vi "buffer_get.vi"(0 "reference in":refnum<class "OSA.lvclass">, 5 "error in (no error)":errorcluster) -> (13 "spectrum X, (wavenr/cm)":sgl[](array[numeric]), 14 "reference out":refnum<class "OSA.lvclass">, 15 "interferogram (16bit)":sgl[](array[numeric]), 16 "interferogram prop":T3 {"contrast" format="%.2f"; "OPDmax (cm)" format="%.2f"; "OPDmin (cm)" format="%.2f"; "peakToPeak position (cm)" format="%.2f"; "peakToPeak, (counts)" format="%.2f"; "X max (cm)" format="%.2f"; "X min (cm)" format="%.2f"}, 17 "spectrum Y (mW)":sgl[](array[numeric]), 18 "spectrum properties":T2, 19 "error out":errorcluster)   [LabVIEW 2010, in "OSA.lvclass"]
doc: "This vi will read data from a labview interferogram and spectrum buffer. The buffer contains only the latest acquired interferogram and spectrum. Use the trace vis to simultaneously handle several data sets.\n\nInterferogram X data unit: cm\nInterferogram Y data unit: ADC counts, (see specs for nr of bits).\nSpectrum X data unit: /cm\nSpectrum Y data unit: mW\n\nFor some OSA, the Spectrum X array will only contain two values; x-min and max. This is indicated by the X VAL OPTION spectrum property (cluster).\n\nSee converter vis to obtain other units, (Modules Unit Conversion in FTSLib help).\n\nTransfer trace data to labview buffer with trace_toLVBuffer.vi."
uses:
  OSA.lvclass
  typeDef/interferogram_properties.ctl
  typeDef/xVal_option.ctl
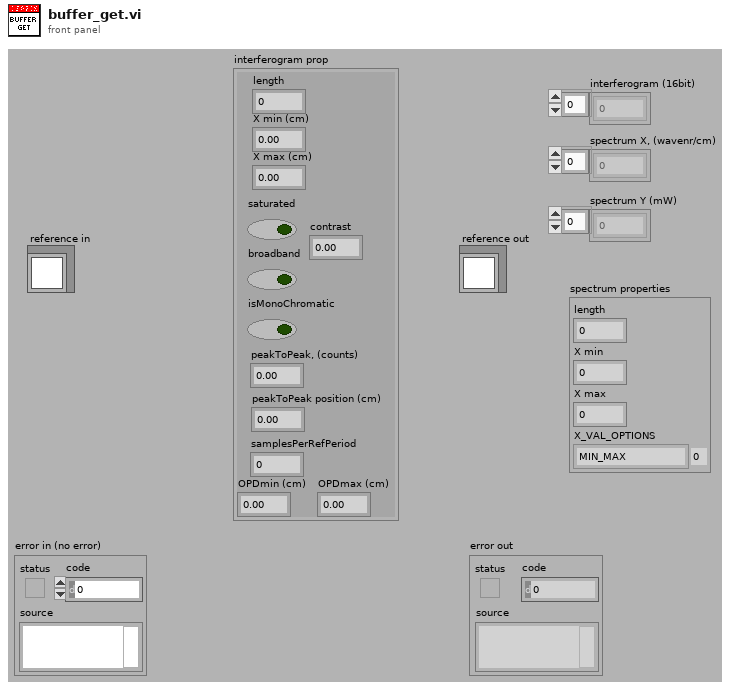
[diagram p1: front panel]
types:
  T1 = typedef "OSA.lvclass/xVal_option.ctl" = enum16{"MIN_MAX", "ARRAY"}
  T2 = cluster{"length":u32, "X min":sgl, "X max":sgl, "X_VAL_OPTIONS":T1}
  T3 = typedef "OSA.lvclass/interferogram_properties.ctl" = cluster{"length":u32, "X min (cm)":sgl, "X max (cm)":sgl, "saturated":bool, "broadband":bool, "isMonoChromatic":bool, "peakToPeak, (counts)":dbl, "peakToPeak position (cm)":dbl, "samplesPerRefPeriod":i32, "OPDmin (cm)":sgl, "OPDmax (cm)":sgl, "contrast":dbl}
  T4 = enum16{"get", "init", "set interferogram", "set spectrum", "cleanUp"}
  T5 = typedef "OSA.lvclass/spectrum_properties.ctl" = cluster{"length":u32, "X min":sgl, "X max":sgl, "X_VAL_OPTIONS":T1}
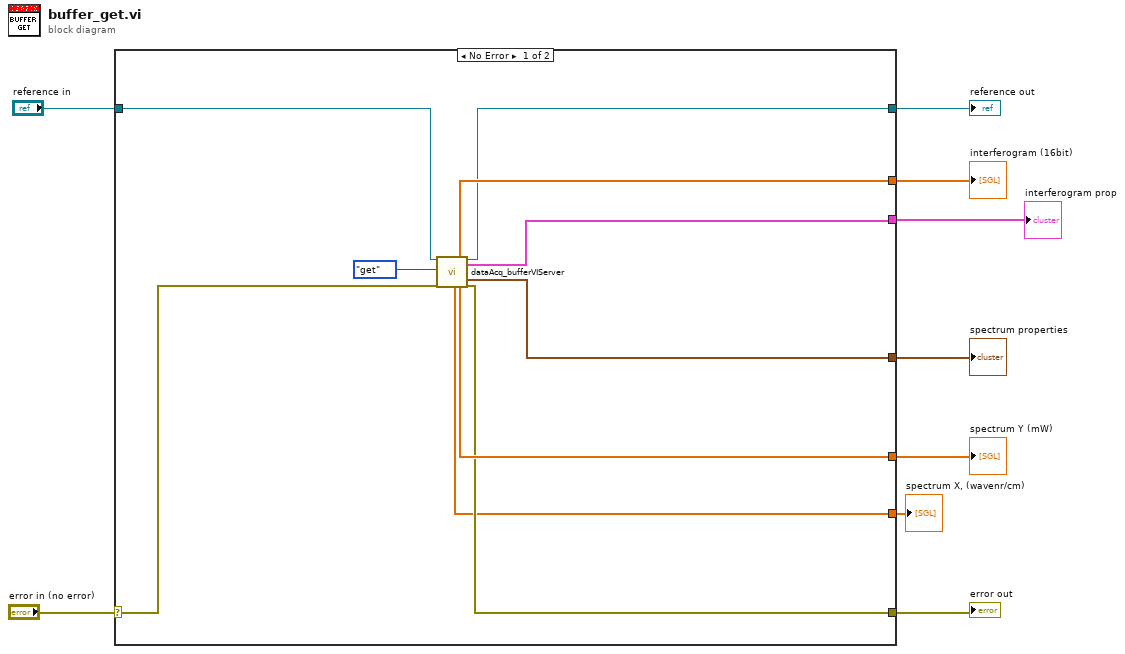
[diagram p0: block diagram]
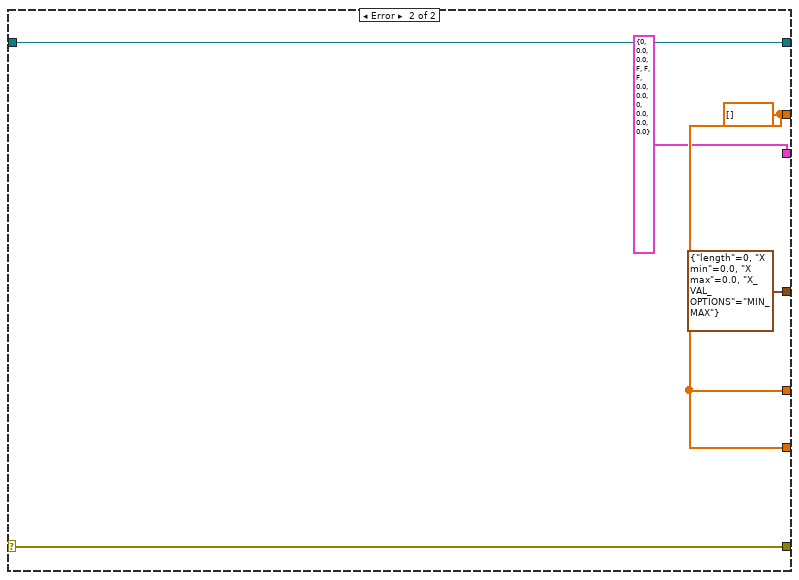
[diagram p2: hidden frame]
diagram:
  n1 = case shown="No Error" "error in (no error)" {
    selector: "error in (no error)" -> [w11 w24]
    tunnel: [w14 w24] -> w8
    tunnel: [w12 w23] -> w6
    tunnel: "reference in" -> [w13 w23]
    tunnel: [w18 w22] -> w5
    tunnel: [w17 w22] -> w3
    tunnel: [w16 T3 {"length"=0, "X min (cm)"=0.0, "X max (cm)"=0.0, "saturated"=FALSE, "broadband"=FALSE, "isMonoChromatic"=FALSE, "peakToPeak, (counts)"=0.0, "peakToPeak position (cm)"=0.0, "samplesPerRefPeriod"=0, "OPDmin (cm)"=0.0, "OPDmax (cm)"=0.0, "contrast"=0.0} ("interferogram prop")] -> w1
    tunnel: [w15 T2 {"length"=0, "X min"=0.0, "X max"=0.0, "X_VAL_OPTIONS"=enum."MIN_MAX"} ("spectrum property")] -> w4
    tunnel: [w10 w22] -> w2
    frame No Error {
      n2 = call "dataAcq_bufferVIServer.vi"("reference"=w13, "action"=T4."get", "error in (no error)"=w11) -> ("spectrum X"=w10:sgl[], "interferogram"=w18:sgl[], "spectrum Y"=w17:sgl[], "duplicate reference"=w12:refnum<class "OSA.lvclass">, "interferogram prop"=w16:T3, "spectrum prop"=w15:T5, "error out"=w14:errorcluster)  [unwired: 9 in, 1 out]
    }
    frame Error {
      w22 = sgl[] [] ("interferogram")
    }
  }
  "error out" <- w8
  "reference out" <- w6
  "interferogram (16bit)" <- w5
  "interferogram prop" <- w1
  "spectrum properties" <- w4
  "spectrum Y (mW)" <- w3
  "spectrum X, (wavenr/cm)" <- w2
